vi "SL TAGS Update Values Into Tags.vi"(8 "error in (no error)":errorcluster, 9 "Tag Update Values":T9[](array[typedef]), 10 "Tag Type":T1, 11 "Tags In":T2[](array[typedef])) -> (0 "error out":errorcluster, 3 "Tags Out":T2[](array[typedef]))   [LabVIEW 2017, in "EEISysLink.lvclass"]
doc: "Where names match update tags with the value input in tag values. \n\nJames Tillett P.E.\nEndeavor Engineering Inc.\nwww.endeavoreng.com"
uses:
  EEISysLink.lvclass
  Controls/SL Tag.ctl
  <vilib>/Skyline/Tag/Wrapper/Wrapper_class/NI Skyline Tag.lvclass
  Controls/SL Tag Properties.ctl
  Controls/SL Tag Data Type.ctl
  Controls/SL Tag Interpolation Method.ctl
  Controls/SL Tag Unit of Measure.ctl
  Controls/SL Tag Type.ctl
  <vilib>/Skyline/Tag/Shared/typedefs/Tag Cluster.ctl
  <vilib>/Skyline/Tag/Shared/typedefs/DataType.ctl
  Controls/SL Tag Value.ctl
  <vilib>/Skyline/Tag/Shared/NI Skyline Tag.lvlib
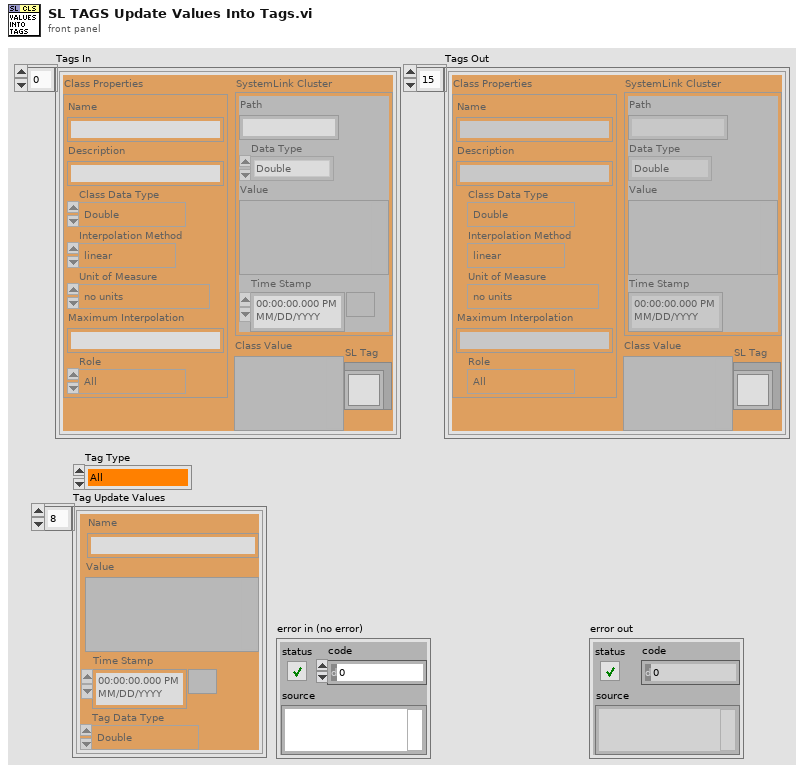
[diagram p1: front panel]
types:
  T1 = typedef "EEISysLink.lvclass/SL Tag Type.ctl" = enum16{"All", "Supervisor", "Worker"}
  T2 = typedef "EEISysLink.lvclass/SL Tag.ctl" = cluster{"Class Properties":T3, "SL Tag":refnum<class "NI Skyline Tag.lvclass">, "SystemLink Cluster":T7, "Class Value":variant}
  T3 = typedef "EEISysLink.lvclass/SL Tag Properties.ctl" = cluster{"Class Data Type":T4, "Name":string, "Description":string, "Interpolation Method":T5, "Unit of Measure":T6, "Maximum Interpolation":string, "Role":T1}
  T4 = typedef "EEISysLink.lvclass/SL Tag Data Type.ctl" = enum16{"Double", "Integer", "String", "Boolean", "Waveform"}
  T5 = typedef "EEISysLink.lvclass/SL Tag Interpolation Method.ctl" = enum16{"linear", "pilinear", "step"}
  T6 = typedef "EEISysLink.lvclass/SL Tag Unit of Measure.ctl" = enum16{"no units", "Second", "Hour", "Minute", "Day", "Year", "Month", "Week", "Foot", "Yard", "Meter", "Centimeter", "Inch", "Mile", "Nautical Mile", "Miles per Hour", "Meters per second", "Square meter", "Cubic meter", "Cubic centimeter", "Cubic inch", "Liter", "Gallon", "Gallons dry US", "Gallon UK", "Percent", "Revolutions per minute", "Revolution", "Degree angle", "Astronomical Unit", "Atom", "Atomic mass", "Bar", "Byte", "C (speed of light)", "Curie", "Decibel", "Electron Volt", "Ounce", "Knot", "G", "Grade", "Are", "Hectare", "Faraday", "Franklin", "Gilbert", "Erg", "Lambert", "Maxwell", "Gauss", "Electron mass", "Kilogram force", "Pound force", "Rad", "Centiradian", "Sphere", "Mach", "Fluid Ounces", "Fluid Ounces UK", "Fahrenheit", "Celsius", "Kelvin", "Rankine", "Gram", "Kilogram", "Pound", "Short/US Ton", "Long/UK ton", "Metric ton", "Mole", "Pounds per square inch", "Inches water column", "Torr", "Millitorr", "Millimeter mercury", "Inches mercury", "Bar (2)", "Atmosphere", "Pascal", "Watt", "kiloWatt", "Horsepower", "Kilowatt Hour", "British thermal units", "Millions of BTU", "Ampere", "Candela", "Radian", "Steradian", "Bit", "Hertz", "Newton", "Joule", "Coulomb", "Volt", "Farad", "Ohm", "Siemens", "Weber", "Tesla", "Henry", "Lumen", "Lux", "Becqueral", "Gray", "Sievert", "Katal", "Angstrom", "Light Year", "Parsec", "Point", "Pixel", "Dyne", "Kilogram force (2)", "Pound force (2)", "Rem", "Rutherford", "Roentgen"}
  T7 = typedef "NI Skyline Tag.lvlib/Tag Cluster.ctl" = cluster{"Path":string, "Data Type":T8, "Value":variant, "Time Stamp":timestamp}
  T8 = typedef "NI Skyline Tag.lvlib/DataType.ctl" = enum32{"Double", "Integer", "String"}
  T9 = typedef "SL Tag Value.ctl" = cluster{"Value":variant, "Time Stamp":timestamp, "Tag Data Type":T4, "Name":string}
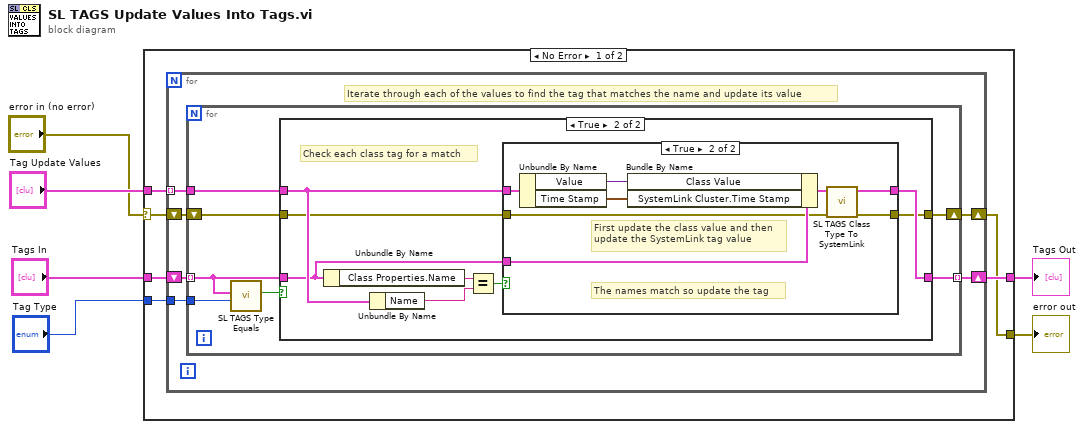
[diagram p0: block diagram]
diagram:
  n1 = case shown="No Error" "error in (no error)" {
    selector: "error in (no error)" -> [w8 w46]
    tunnel: [w12 w47] -> w6
    tunnel: "Tag Update Values" -> [w11 _]
    tunnel: "Tags In" -> [w10 w47]
    tunnel: "Tag Type" -> [w9 _]
    tunnel: [w7 w46] -> w1
    frame No Error {
      n2 = for {
        tunnel: w11 -> [w16] mode=indexing
        shift-right: [w17] -> w12
        shift-left: w10 -> [w18]
        tunnel: w9 -> [w15]
        shift-right: [w13] -> w7
        shift-left: w8 -> [w14]
        # "Iterate through each of the values to find the tag that matches the name and update its value"
        n3 = for {
          tunnel: w18 -> [w23] mode=indexing
          tunnel: w16 -> [w24]
          tunnel: [w25] -> w17 mode=indexing
          tunnel: w15 -> [w22]
          shift-right: [w19] -> w13
          shift-left: w14 -> [w20]
          n4 = call "SL TAGS Type Equals.vi"("Tag Type"=w22, "Tag"=w23) -> ("Match?"=w21:bool)  [unwired: 9 in]
          n5 = case shown="True" w21 {
            tunnel: [w27 w34] -> w25
            tunnel: w24 -> [_ w33]
            tunnel: w23 -> [w27 w31]
            tunnel: w20 -> [w26 w29]
            tunnel: [w26 w30] -> w19
            frame False {
            }
            frame True {
              # "Check each class tag for a match"
              n6 = Unbundle By Name(w31) -> ("Class Properties.Name"=w35:string)
              n7 = Unbundle By Name(w33) -> ("Name"=w32:string)
              n8 = Equal?(x=w35, y=w32) -> (x = y?=w28:bool)
              n9 = case shown="True" w28 {
                tunnel: w33 -> [_ w43]
                tunnel: w31 -> [w37 w42]
                tunnel: [w37 w40] -> w34
                tunnel: [w36 w38] -> w30
                tunnel: w29 -> [w36 w39]
                frame False {
                  # "Names don't match so do nothing"
                }
                frame True {
                  # "First update the class value and then\nupdate the SystemLink tag value"
                  # "The names match so update the tag"
                  n10 = Unbundle By Name(w43) -> ("Value"=w44:variant, "Time Stamp"=w45:timestamp)
                  n11 = Bundle By Name(cluster=w42, "Class Value"=w44, "SystemLink Cluster.Time Stamp"=w45) -> (w41:T2)
                  n12 = call "SL TAGS Class Type To SystemLink.vi"("error in (no error)"=w39, "Class Tag In"=w41) -> ("error out"=w38:errorcluster, "Class Tag Out"=w40:T2)  [unwired: 7 in, 1 out]
                }
              }
            }
          }
        }
      }
    }
    frame Error {
    }
  }
  "Tags Out" <- w6
  "error out" <- w1
